vi "autoSelectData.vi"(9 "command and parameters in":string[](array[string]), 10 "index":u8, 11 "sensor datas":T1) -> (2 "accessed value":dbl)   [LabVIEW 2012]
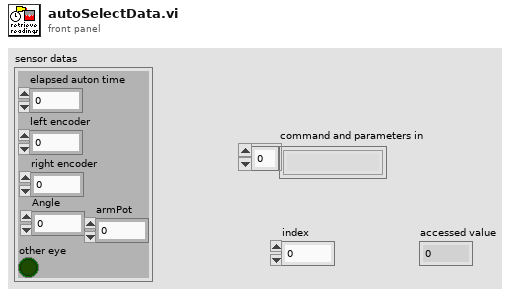
[diagram p1: front panel]
types:
  T1 = cluster{"elapsed auton time":dbl, "left encoder":dbl, "other eye":bool, "right encoder":dbl, "Angle":dbl, "armPot":dbl}
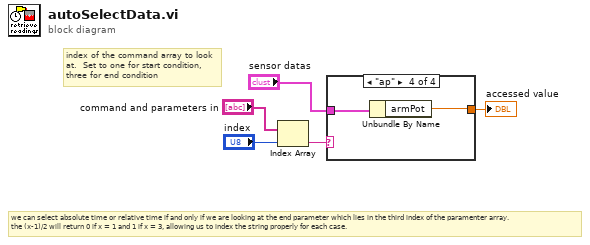
[diagram p0: block diagram]
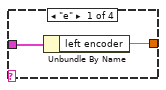
[diagram p2: hidden frame]
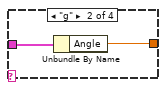
[diagram p3: hidden frame]
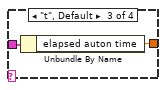
[diagram p4: hidden frame]
diagram:
  # "we can select absolute time or relative time if and only if we are looking at the end parameter which lies in the third index of the paramenter array.\nthe (x-1)/2 will return 0 if x = 1 and 1 if x = 3, allowing us to index the string properly for each case."
  # "index of the command array to look at.  Set to one for start condition, three for end condition"
  n1 = Index Array(array="command and parameters in", index="index") -> (element=w3:string)
  n2 = case shown="\"ap\"" w3 {
    tunnel: "sensor datas" -> [w7 w9 w11 w13]
    tunnel: [w6 w8 w10 w12] -> w4
    frame "e" {
      n3 = Unbundle By Name(w7) -> ("left encoder"=w6:dbl)
    }
    frame "g" {
      n4 = Unbundle By Name(w9) -> ("Angle"=w8:dbl)
    }
    frame "t", Default {
      n5 = Unbundle By Name(w11) -> ("elapsed auton time"=w10:dbl)
    }
    frame "ap" {
      n6 = Unbundle By Name(w13) -> ("armPot"=w12:dbl)
    }
  }
  "accessed value" <- w4
